vi "Main.vi"(8 "error in (no error)":errorcluster, 11 "ConfocalStage in":refnum<class "ConfocalStage.lvclass">) -> (0 "error out":errorcluster, 3 "component":refnum<class "ConfocalStage.lvclass">)   [LabVIEW 2012, in "ConfocalStage.lvclass"]
doc: "Main VI of the component. This should contain the GUI of your component and be called when creating an executable."
uses:
  ConfocalStage.lvclass
  <vilib>/Distrio/Murmex/Murmex/command_enum.ctl
  <vilib>/Distrio/Murmex/InitialiseMessage/InitialiseMessage.lvclass
  <vilib>/Distrio/Murmex/ConfigureMessage/ConfigureMessage.lvclass
  <vilib>/Distrio/Murmex/TerminateMessage/TerminateMessage.lvclass
  <vilib>/Distrio/Murmex/GenericMessage/GenericMessage.lvclass
  ConfocalStage.lvclass/ConfocalStage.ctl
  <vilib>/Distrio/Murmex/Murmex/Murmex.lvclass
  <vilib>/Distrio/Murmex/Murmex/Set configure at initialise.vi
  <vilib>/Distrio/Murmex/Murmex/Set log reference.vi
  <vilib>/Distrio/Murmex/Murmex/Set VI reference.vi
  <vilib>/Distrio/Murmex/Murmex/Get ID.vi
  <vilib>/Distrio/Murmex/Murmex/Set write log to disk.vi
  <vilib>/Distrio/Murmex/Message/Message.lvclass
panel:
  in  "button:quit":bool
  in  "button:configure":bool
  in  "terminate?":bool
  in  "Tab Control":enum32{"User", "Debug"}(tab)
  in  "focus step":dbl
  in  "Y step":dbl
  in  "X step":dbl
  in  "button:focus_forward":bool
  in  "button:focus_backward":bool
  in  "button:Y_forward":bool
  in  "button:Y_backward":bool
  in  "button:X_forward":bool
  in  "button:X_backward":bool
  in  "button:set as focus max":bool
  in  "button:set as Y max":bool
  in  "button:set as X max":bool
  in  "button:set as focus min":bool
  in  "button:set as Y min":bool
  in  "button:set as X min":bool
  in  "button:set as origin":bool
  in  "X position":dbl
  in  "Y position":dbl
  in  "focus position":dbl
  out "out of limits?":bool
  in  "Component id":string="ConfStage"
  in  "button:send command":bool
  in  "command":T1
  in  "generic command":string
  out "log":string
  # "Position"
  # "Step size"
  # "X"
  # "Y"
  # "Focus"
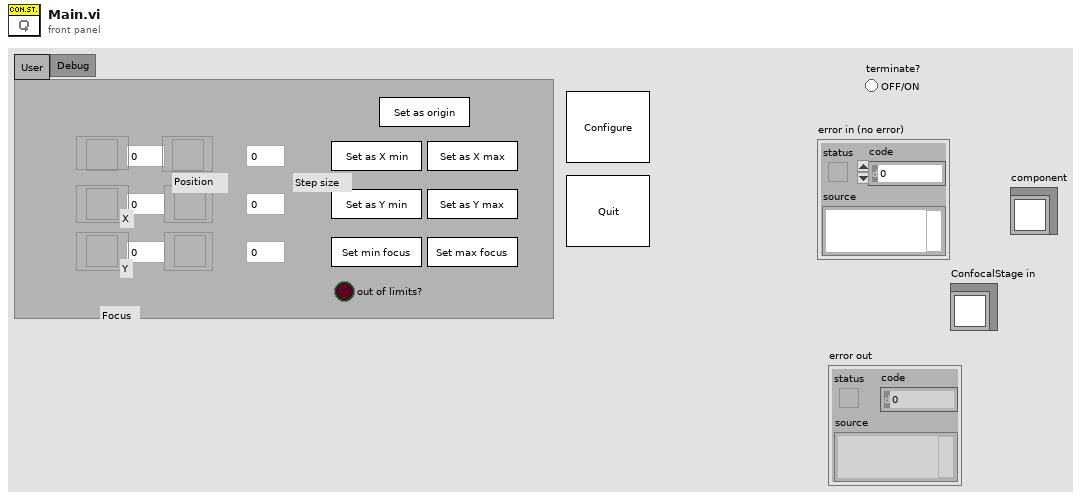
[diagram p1: front panel]
types:
  T1 = typedef "Murmex.lvlib/Murmex.lvclass/command_enum.ctl" = enum16{"null", "initialise", "reset", "terminate", "acknowledge", "update", "inspect", "inform", "proceed", "start", "stop", "fetch", "configure", "generic"}
  T2 = enum8{"Enabled", "Disabled", "Disabled and Grayed Out"}
  T3 = typedef "Murmex.lvclass/command_enum.ctl" = enum16{"null", "initialise", "reset", "terminate", "acknowledge", "update", "inspect", "inform", "proceed", "start", "stop", "fetch", "configure", "generic"}
  T4 = typedef "Murmex.lvclass/Event type enumerations.ctl" = enum16{"before", "after"}
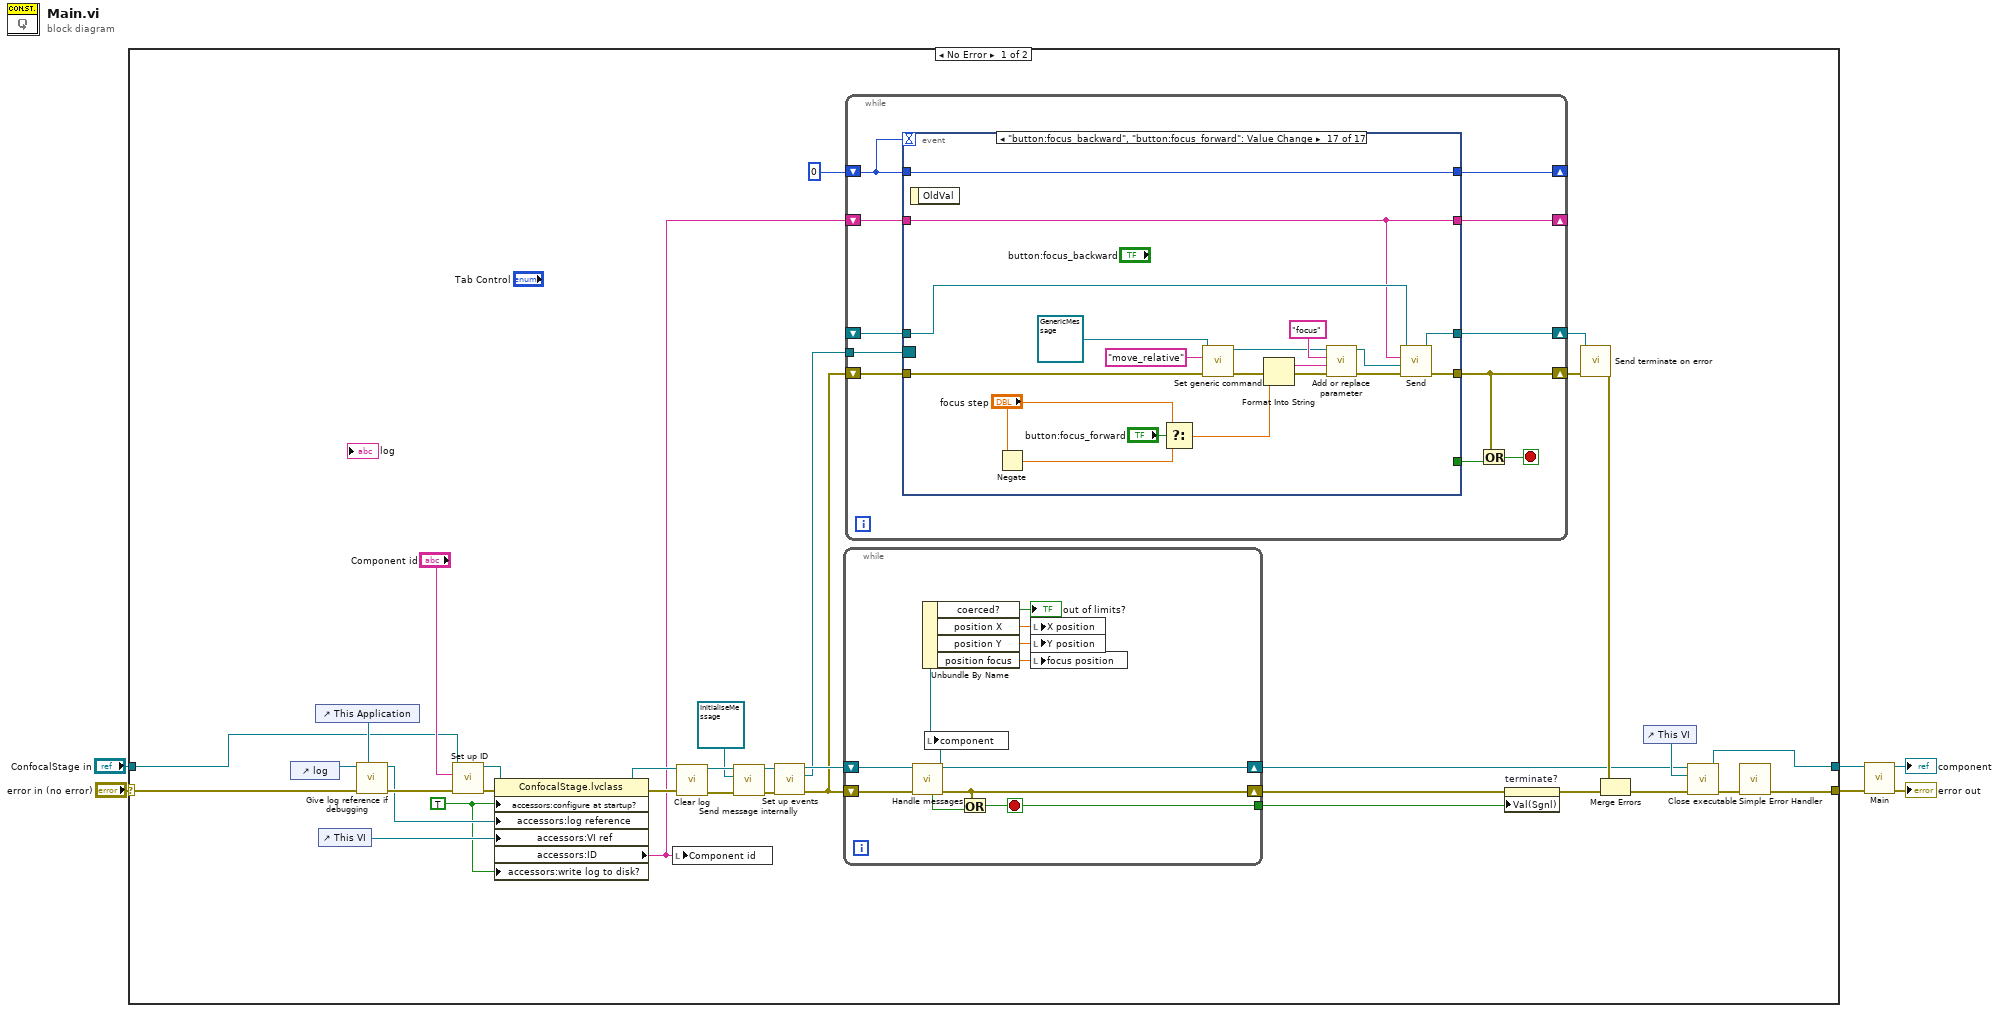
[diagram p0: block diagram]
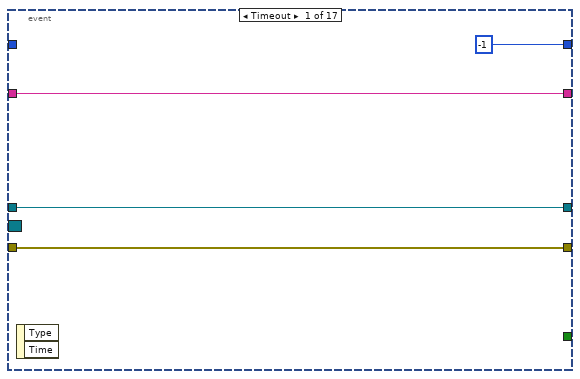
[diagram p2: hidden frame]
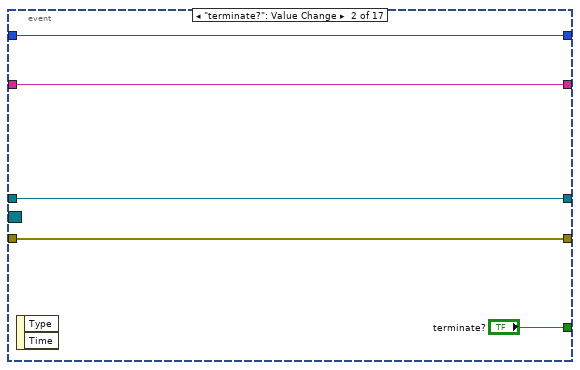
[diagram p3: hidden frame]
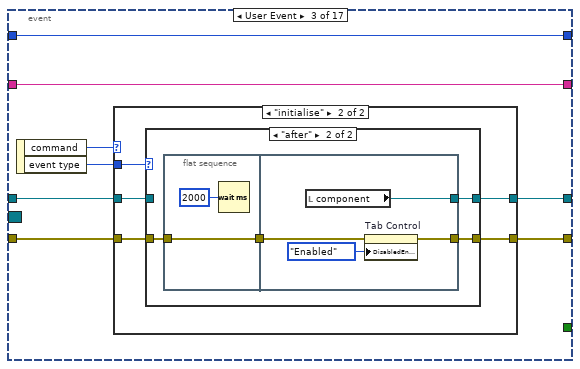
[diagram p4: hidden frame]
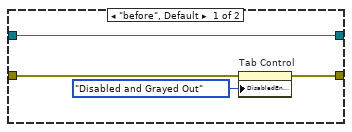
[diagram p6: hidden frame]
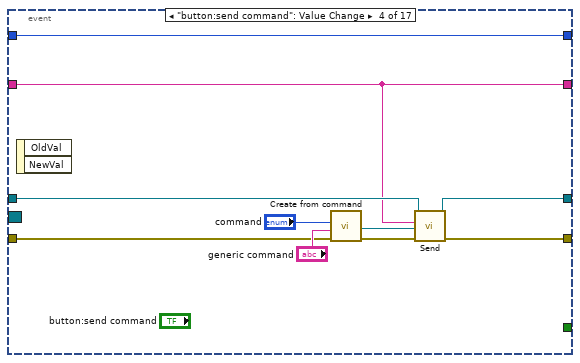
[diagram p7: hidden frame]
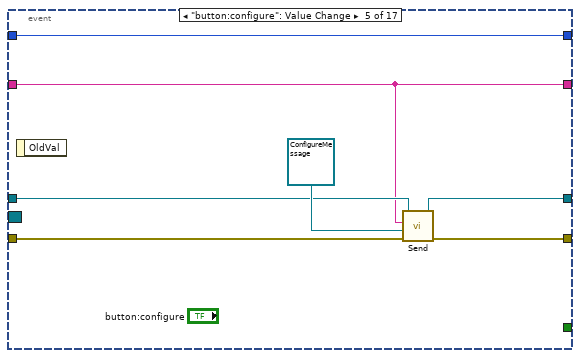
[diagram p8: hidden frame]
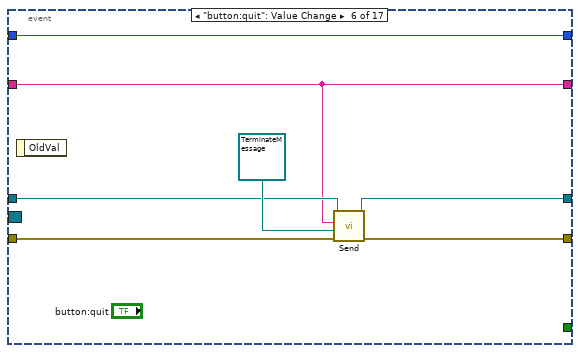
[diagram p9: hidden frame]
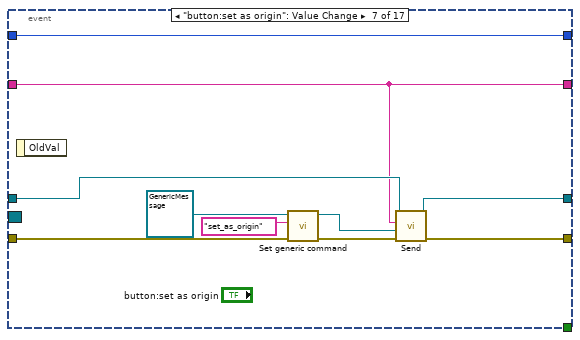
[diagram p10: hidden frame]
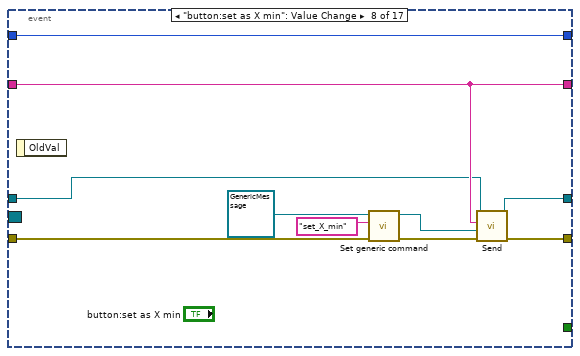
[diagram p11: hidden frame]
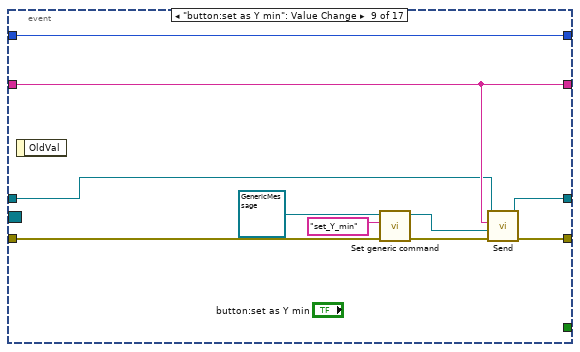
[diagram p12: hidden frame]
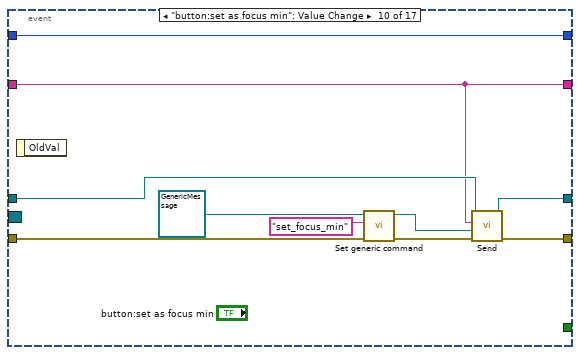
[diagram p13: hidden frame]
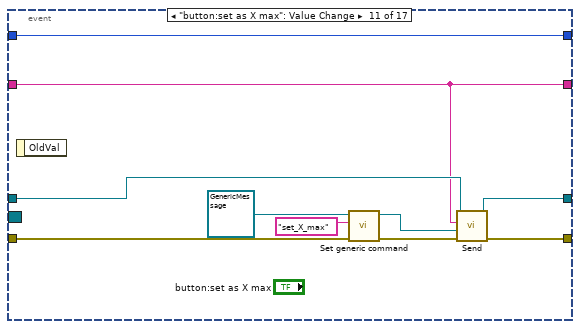
[diagram p14: hidden frame]
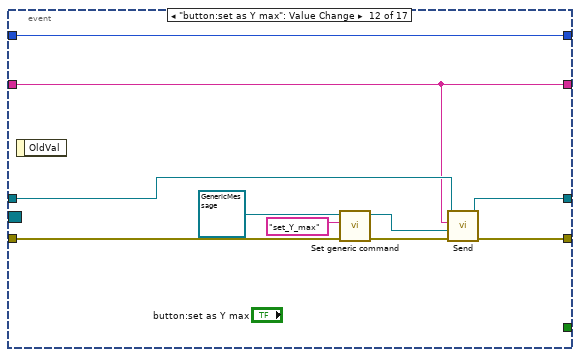
[diagram p15: hidden frame]
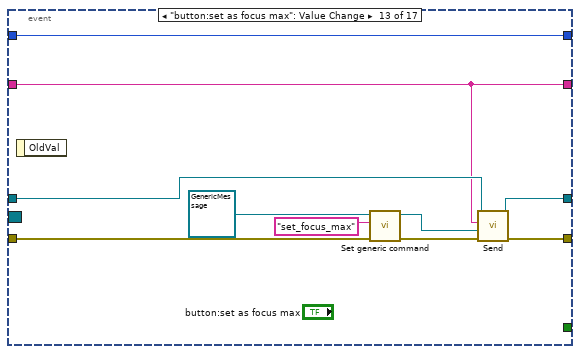
[diagram p16: hidden frame]
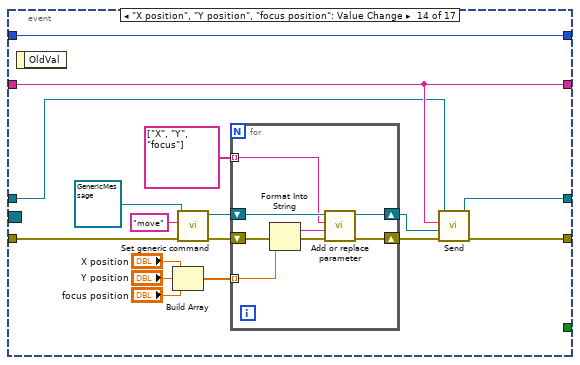
[diagram p17: hidden frame]
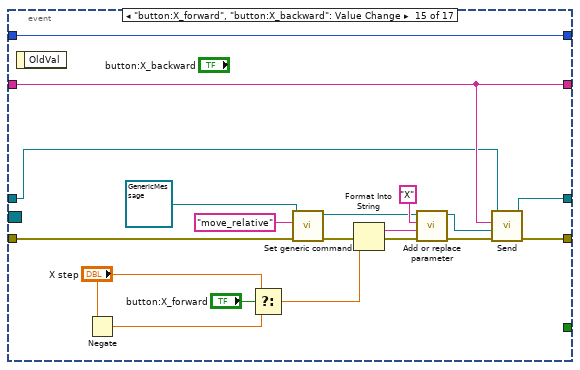
[diagram p18: hidden frame]
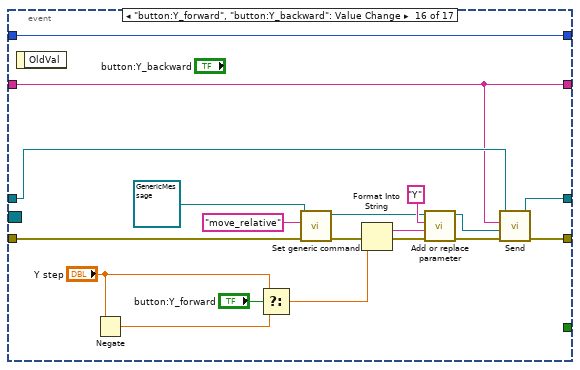
[diagram p19: hidden frame]
diagram:
  n1 = case shown="No Error" "error in (no error)" {
    selector: "error in (no error)" -> [w26 w278]
    tunnel: [w14 w278] -> w3
    tunnel: [w13 w277] -> w2
    tunnel: "ConfocalStage in" -> [w25 w277]
    frame No Error {
      w7 = TRUE ("configure at startup?")
      n2 = control-ref of="log"() -> (w35:refnum<vi>)
      n3 = control-ref of="This Application"() -> (w41:refnum<vi>)
      n4 = control-ref of="This VI"() -> (w34:refnum<vi>)
      n5 = call "Give log reference if debugging.vi"("application ref"=w41, "error in (no error)"=w26, "log reference in"=w35) -> ("error out"=w40:errorcluster, "log reference out"=w36:refnum<vi>)  [unwired: 6 in, 1 out]
      n6 = call <vilib>:"Set up ID.vi"("error in (no error)"=w40, "component ID"="Component id", "MurmexBase in"=w25) -> ("error out"=w38:errorcluster, "MurmexBase out"=w37:refnum<class "ConfocalStage.lvclass">)  [unwired: 6 in, 1 out]
      n7 = property class="ConfocalStage.lvclass"(reference=w37, error in=w38, "accessors:configure at startup?"=w7, "accessors:log reference"=w36, "accessors:VI ref"=w34, "accessors:write log to disk?"=w7) -> (reference out=w27:refnum<class "ConfocalStage.lvclass">, error out=w29:errorcluster, "accessors:ID"=w22:string)
      n8 = local write "Component id"(w22) -> ()
      n9 = call <vilib>:"Clear log.vi"("error in (no error)"=w29, "MurmexBase in"=w27) -> ("error out"=w32:errorcluster, "MurmexBase out"=w33:refnum<class "ConfocalStage.lvclass">)  [unwired: 8 in]
      n10 = call <vilib>:"Send message internally.vi"("error in (no error)"=w32, "Message"=refnum<class "InitialiseMessage.lvclass"> refnum ("InitialiseMessage"), "Murmex in"=w33) -> ("error out"=w31:errorcluster, "Murmex out"=w30:refnum<class "ConfocalStage.lvclass">)  [unwired: 7 in]
      n11 = call <vilib>:"Set up events.vi"("error in (no error)"=w31, "MurmexBase in"=w30) -> ("error out"=w23:errorcluster, "Event Registration Refnum"=w21:refnum<event-registration>, "MurmexBase out"=w24:refnum<class "ConfocalStage.lvclass">)  [unwired: 7 in]
      n12 = while {
        shift-right: [w271] -> w15
        shift-left: w24 -> [w274]
        shift-right: [w273] -> w12
        shift-left: w23 -> [w275]
        tunnel: [w272] -> w10
        stop <- w272 stop-if-true
        n13 = call <vilib>:"Handle messages.vi"("error in (no error)"=w275, "Murmex in"=w274) -> ("error out"=w273:errorcluster, "Murmex out"=w271:refnum<class "ConfocalStage.lvclass">, "terminated?"=w276:bool)  [unwired: 7 in]
        n14 = Unbundle By Name(w271) -> ("coerced?"=→"out of limits?":bool, "position X"=w270:dbl, "position Y"=w269:dbl, "position focus"=w268:dbl)
        n15 = local write "component"(w271) -> ()
        n16 = Or(x=w273, y=w276) -> (x .or. y?=w272:bool)
        n17 = local write "X position"(w270) -> ()
        n18 = local write "Y position"(w269) -> ()
        n19 = local write "focus position"(w268) -> ()
      }
      n20 = while {
        shift-right: [w45] -> w9
        shift-left: w23 -> [w49]
        shift-right: [w48] -> _
        shift-left: w22 -> [w47]
        tunnel: w21 -> [w52]
        shift-right: [w50] -> _
        shift-left: 0 -> [w51]
        shift-right: [w43] -> w8
        shift-left: _ -> [w42]
        stop <- w44 stop-if-true
        n21 = event shown="[16] \"button:focus_backward\", \"button:focus_forward\": Value Change" {
          selector: w52 -> [_ _ _ _ _ _ _ _ _ _ _ _ _ _ _ _ _]
          dyn-events: _ -> [_ _ _ _ _ _ _ _ _ _ _ _ _ _ _ _ _]
          timeout: w51 -> [_ _ _ _ _ _ _ _ _ _ _ _ _ _ _ _ _]
          tunnel: w51 -> [_ w61 w69 w91 w101 w109 w115 w127 w137 w146 w155 w165 w175 w187 w213 w232 w250]
          tunnel: [-1 w61 w69 w91 w101 w109 w115 w127 w137 w146 w155 w165 w175 w187 w213 w232 w250] -> w50
          tunnel: [w55 w59 w65 w95 w105 w112 w120 w129 w139 w149 w159 w169 w180 w190 w215 w236 w254] -> w45
          tunnel: w49 -> [w55 w59 w66 w96 w106 w113 w122 w130 w140 w150 w160 w170 w179 w195 w219 w235 w255]
          tunnel: [w54 w60 w62 w93 w103 w108 w116 w128 w138 w147 w156 w166 w176 w188 w214 w233 w251] -> w48
          tunnel: w47 -> [w54 w60 w62 w93 w103 w108 w116 w128 w138 w147 w156 w166 w176 w188 w214 w233 w251]
          tunnel: [_ "terminate?" _ _ _ _ _ _ _ _ _ _ _ _ _ _ _] -> w46
          tunnel: [w53 w57 w64 w92 w102 w110 w117 w125 w135 w145 w157 w167 w177 w185 w211 w231 w252] -> w43
          tunnel: w42 -> [w53 w57 w63 w94 w104 w111 w118 w126 w136 w148 w158 w168 w178 w186 w212 w234 w253]
          event Timeout {
            n22 = event-data() -> ()  [unwired: 1 in, 2 out]
          }
          event "terminate?": Value Change {
            n23 = event-data() -> ()  [unwired: 1 in, 2 out]
          }
          event User Event {
            n24 = event-data() -> ("command"=w68:T3, "event type"=w67:T4)  [unwired: 1 in]
            n25 = case shown="\"initialise\"" w68 {
              tunnel: w67 -> [_ w76]
              tunnel: w66 -> [w70 w75]
              tunnel: [w70 w74] -> w65
              tunnel: [w71 w73] -> w64
              tunnel: w63 -> [w71 w72]
              frame "null", Default {
              }
              frame "initialise" {
                n26 = case shown="\"after\"" w76 {
                  tunnel: w75 -> [w80 w83]
                  tunnel: [w79 w82] -> w74
                  tunnel: [w77 w81] -> w73
                  tunnel: w72 -> [w77 _]
                  frame "before", Default {
                    n27 = property on="Tab Control" class="TabCtl (strict)"(error in=w80, "DisabledEnum"=T2."Disabled and Grayed Out" ("Disabled")) -> (error out=w79:errorcluster)  [unwired: 1 in, 1 out]
                  }
                  frame "after" {
                    n28 = flat-sequence {
                      tunnel: [w85] -> w84
                      tunnel: w83 -> [w85]
                      tunnel: w84 -> [w89]
                      tunnel: [w88] -> w82
                      tunnel: [w87] -> w81
                      frame #0 {
                        n29 = Wait (ms)(milliseconds to wait=u32 2000) -> ()  [unwired: 1 out]
                      }
                      frame #1 {
                        n30 = local read "component"() -> (w87:refnum<class "ConfocalStage.lvclass">)
                        n31 = property on="Tab Control" class="TabCtl (strict)"(error in=w89, "DisabledEnum"=T2."Enabled" ("Disabled")) -> (error out=w88:errorcluster)  [unwired: 1 in, 1 out]
                      }
                    }
                  }
                }
              }
            }
          }
          event "button:send command": Value Change {
            n32 = event-data() -> ()  [unwired: 1 in, 2 out]
            n33 = call <vilib>:"Create from command.vi"("error in (no error)"=w96, "generic command"="generic command", "command"="command") -> ("error out"=w97:errorcluster, "Message out"=w100:refnum<class "Message.lvclass">)  [unwired: 7 in]
            n34 = call <vilib>:"Send.vi"("error in (no error)"=w97, "Message"=w100, "recipient"=w93, "Murmex in"=w94) -> ("error out"=w95:errorcluster, "Murmex out"=w92:refnum<class "ConfocalStage.lvclass">)  [unwired: 6 in]
          }
          event "button:configure": Value Change {
            n35 = event-data() -> ()  [unwired: 1 in, 1 out]
            n36 = call <vilib>:"Send.vi"("error in (no error)"=w106, "Message"=refnum<class "ConfigureMessage.lvclass"> refnum ("ConfigureMessage"), "recipient"=w103, "Murmex in"=w104) -> ("error out"=w105:errorcluster, "Murmex out"=w102:refnum<class "ConfocalStage.lvclass">)  [unwired: 6 in]
          }
          event "button:quit": Value Change {
            n37 = event-data() -> ()  [unwired: 1 in, 1 out]
            n38 = call <vilib>:"Send.vi"("error in (no error)"=w113, "Message"=refnum<class "TerminateMessage.lvclass"> refnum ("TerminateMessage"), "recipient"=w108, "Murmex in"=w111) -> ("error out"=w112:errorcluster, "Murmex out"=w110:refnum<class "ConfocalStage.lvclass">)  [unwired: 6 in]
          }
          event "button:set as origin": Value Change {
            n39 = event-data() -> ()  [unwired: 1 in, 1 out]
            n40 = call <vilib>:"Set generic command.vi"("error in (no error)"=w122, "generic command"="set_as_origin", "GenericMessage in"=refnum<class "GenericMessage.lvclass"> refnum ("Message in")) -> ("error out"=w121:errorcluster, "GenericMessage out"=w119:refnum<class "GenericMessage.lvclass">)  [unwired: 7 in]
            n41 = call <vilib>:"Send.vi"("error in (no error)"=w121, "Message"=w119, "recipient"=w116, "Murmex in"=w118) -> ("error out"=w120:errorcluster, "Murmex out"=w117:refnum<class "ConfocalStage.lvclass">)  [unwired: 6 in]
          }
          event "button:set as X min": Value Change {
            n42 = event-data() -> ()  [unwired: 1 in, 1 out]
            n43 = call <vilib>:"Set generic command.vi"("error in (no error)"=w130, "generic command"="set_X_min", "GenericMessage in"=refnum<class "GenericMessage.lvclass"> refnum ("Message in")) -> ("error out"=w133:errorcluster, "GenericMessage out"=w134:refnum<class "GenericMessage.lvclass">)  [unwired: 7 in]
            n44 = call <vilib>:"Send.vi"("error in (no error)"=w133, "Message"=w134, "recipient"=w128, "Murmex in"=w126) -> ("error out"=w129:errorcluster, "Murmex out"=w125:refnum<class "ConfocalStage.lvclass">)  [unwired: 6 in]
          }
          event "button:set as Y min": Value Change {
            n45 = event-data() -> ()  [unwired: 1 in, 1 out]
            n46 = call <vilib>:"Set generic command.vi"("error in (no error)"=w140, "generic command"="set_Y_min", "GenericMessage in"=refnum<class "GenericMessage.lvclass"> refnum ("Message in")) -> ("error out"=w142:errorcluster, "GenericMessage out"=w141:refnum<class "GenericMessage.lvclass">)  [unwired: 7 in]
            n47 = call <vilib>:"Send.vi"("error in (no error)"=w142, "Message"=w141, "recipient"=w138, "Murmex in"=w136) -> ("error out"=w139:errorcluster, "Murmex out"=w135:refnum<class "ConfocalStage.lvclass">)  [unwired: 6 in]
          }
          event "button:set as focus min": Value Change {
            n48 = event-data() -> ()  [unwired: 1 in, 1 out]
            n49 = call <vilib>:"Set generic command.vi"("error in (no error)"=w150, "generic command"="set_focus_min", "GenericMessage in"=refnum<class "GenericMessage.lvclass"> refnum ("Message in")) -> ("error out"=w152:errorcluster, "GenericMessage out"=w151:refnum<class "GenericMessage.lvclass">)  [unwired: 7 in]
            n50 = call <vilib>:"Send.vi"("error in (no error)"=w152, "Message"=w151, "recipient"=w147, "Murmex in"=w148) -> ("error out"=w149:errorcluster, "Murmex out"=w145:refnum<class "ConfocalStage.lvclass">)  [unwired: 6 in]
          }
          event "button:set as X max": Value Change {
            n51 = event-data() -> ()  [unwired: 1 in, 1 out]
            n52 = call <vilib>:"Set generic command.vi"("error in (no error)"=w160, "generic command"="set_X_max", "GenericMessage in"=refnum<class "GenericMessage.lvclass"> refnum ("Message in")) -> ("error out"=w162:errorcluster, "GenericMessage out"=w161:refnum<class "GenericMessage.lvclass">)  [unwired: 7 in]
            n53 = call <vilib>:"Send.vi"("error in (no error)"=w162, "Message"=w161, "recipient"=w156, "Murmex in"=w158) -> ("error out"=w159:errorcluster, "Murmex out"=w157:refnum<class "ConfocalStage.lvclass">)  [unwired: 6 in]
          }
          event "button:set as Y max": Value Change {
            n54 = event-data() -> ()  [unwired: 1 in, 1 out]
            n55 = call <vilib>:"Set generic command.vi"("error in (no error)"=w170, "generic command"="set_Y_max", "GenericMessage in"=refnum<class "GenericMessage.lvclass"> refnum ("Message in")) -> ("error out"=w172:errorcluster, "GenericMessage out"=w171:refnum<class "GenericMessage.lvclass">)  [unwired: 7 in]
            n56 = call <vilib>:"Send.vi"("error in (no error)"=w172, "Message"=w171, "recipient"=w166, "Murmex in"=w168) -> ("error out"=w169:errorcluster, "Murmex out"=w167:refnum<class "ConfocalStage.lvclass">)  [unwired: 6 in]
          }
          event "button:set as focus max": Value Change {
            n57 = event-data() -> ()  [unwired: 1 in, 1 out]
            n58 = call <vilib>:"Set generic command.vi"("error in (no error)"=w179, "generic command"="set_focus_max", "GenericMessage in"=refnum<class "GenericMessage.lvclass"> refnum ("Message in")) -> ("error out"=w182:errorcluster, "GenericMessage out"=w181:refnum<class "GenericMessage.lvclass">)  [unwired: 7 in]
            n59 = call <vilib>:"Send.vi"("error in (no error)"=w182, "Message"=w181, "recipient"=w176, "Murmex in"=w178) -> ("error out"=w180:errorcluster, "Murmex out"=w177:refnum<class "ConfocalStage.lvclass">)  [unwired: 6 in]
          }
          event "X position", "Y position", "focus position": Value Change {
            n60 = event-data() -> ()  [unwired: 1 in, 1 out]
            n61 = Build Array("X position", "Y position", "focus position") -> (w198:dbl[])
            n62 = call <vilib>:"Set generic command.vi"("error in (no error)"=w195, "generic command"="move", "GenericMessage in"=refnum<class "GenericMessage.lvclass"> refnum ("Message in")) -> ("error out"=w194:errorcluster, "GenericMessage out"=w193:refnum<class "GenericMessage.lvclass">)  [unwired: 7 in]
            n63 = for {
              tunnel: w198 -> [w203] mode=indexing
              shift-right: [w204] -> w191
              shift-left: w194 -> [w208]
              shift-right: [w205] -> w189
              shift-left: w193 -> [w206]
              tunnel: string[] ["X", "Y", "focus"] -> [w202] mode=indexing
              n64 = Format Into String(error in=w208, w203) -> (resulting string=w209:string, error out=w207:errorcluster)  [unwired: 2 in]
              n65 = call <vilib>:"Add or replace parameter.vi"("error in (no error)"=w207, "value"=w209, "name"=w202, "Message in"=w206) -> ("error out"=w204:errorcluster, "Message out"=w205:refnum<class "GenericMessage.lvclass">)  [unwired: 6 in]
            }
            n66 = call <vilib>:"Send.vi"("error in (no error)"=w191, "Message"=w189, "recipient"=w188, "Murmex in"=w186) -> ("error out"=w190:errorcluster, "Murmex out"=w185:refnum<class "ConfocalStage.lvclass">)  [unwired: 6 in]
          }
          event "button:X_forward", "button:X_backward": Value Change {
            n67 = event-data() -> ()  [unwired: 1 in, 1 out]
            n68 = Negate(x="X step") -> (-x=w226:dbl)
            n69 = Select(t="X step", s="button:X_forward", f=w226) -> (s? t:f=w210:dbl)
            n70 = call <vilib>:"Set generic command.vi"("error in (no error)"=w219, "generic command"="move_relative", "GenericMessage in"=refnum<class "GenericMessage.lvclass"> refnum ("Message in")) -> ("error out"=w218:errorcluster, "GenericMessage out"=w221:refnum<class "GenericMessage.lvclass">)  [unwired: 7 in]
            n71 = Format Into String(error in=w218, w210) -> (resulting string=w222:string, error out=w217:errorcluster)  [unwired: 2 in]
            n72 = call <vilib>:"Add or replace parameter.vi"("error in (no error)"=w217, "value"=w222, "name"="X", "Message in"=w221) -> ("error out"=w216:errorcluster, "Message out"=w220:refnum<class "GenericMessage.lvclass">)  [unwired: 6 in]
            n73 = call <vilib>:"Send.vi"("error in (no error)"=w216, "Message"=w220, "recipient"=w214, "Murmex in"=w212) -> ("error out"=w215:errorcluster, "Murmex out"=w211:refnum<class "ConfocalStage.lvclass">)  [unwired: 6 in]
          }
          event "button:Y_forward", "button:Y_backward": Value Change {
            n74 = event-data() -> ()  [unwired: 1 in, 1 out]
            n75 = Negate(x="Y step") -> (-x=w247:dbl)
            n76 = Select(t="Y step", s="button:Y_forward", f=w247) -> (s? t:f=w237:dbl)
            n77 = call <vilib>:"Set generic command.vi"("error in (no error)"=w235, "generic command"="move_relative", "GenericMessage in"=refnum<class "GenericMessage.lvclass"> refnum ("Message in")) -> ("error out"=w240:errorcluster, "GenericMessage out"=w242:refnum<class "GenericMessage.lvclass">)  [unwired: 7 in]
            n78 = Format Into String(error in=w240, w237) -> (resulting string=w243:string, error out=w239:errorcluster)  [unwired: 2 in]
            n79 = call <vilib>:"Add or replace parameter.vi"("error in (no error)"=w239, "value"=w243, "name"="Y", "Message in"=w242) -> ("error out"=w238:errorcluster, "Message out"=w241:refnum<class "GenericMessage.lvclass">)  [unwired: 6 in]
            n80 = call <vilib>:"Send.vi"("error in (no error)"=w238, "Message"=w241, "recipient"=w233, "Murmex in"=w234) -> ("error out"=w236:errorcluster, "Murmex out"=w231:refnum<class "ConfocalStage.lvclass">)  [unwired: 6 in]
          }
          event "button:focus_backward", "button:focus_forward": Value Change {
            n81 = event-data() -> ()  [unwired: 1 in, 1 out]
            n82 = Negate(x="focus step") -> (-x=w266:dbl)
            n83 = Select(t="focus step", s="button:focus_forward", f=w266) -> (s? t:f=w256:dbl)
            n84 = call <vilib>:"Set generic command.vi"("error in (no error)"=w255, "generic command"="move_relative", "GenericMessage in"=refnum<class "GenericMessage.lvclass"> refnum ("Message in")) -> ("error out"=w259:errorcluster, "GenericMessage out"=w261:refnum<class "GenericMessage.lvclass">)  [unwired: 7 in]
            n85 = Format Into String(error in=w259, w256) -> (resulting string=w262:string, error out=w258:errorcluster)  [unwired: 2 in]
            n86 = call <vilib>:"Add or replace parameter.vi"("error in (no error)"=w258, "value"=w262, "name"="focus", "Message in"=w261) -> ("error out"=w257:errorcluster, "Message out"=w260:refnum<class "GenericMessage.lvclass">)  [unwired: 6 in]
            n87 = call <vilib>:"Send.vi"("error in (no error)"=w257, "Message"=w260, "recipient"=w251, "Murmex in"=w253) -> ("error out"=w254:errorcluster, "Murmex out"=w252:refnum<class "ConfocalStage.lvclass">)  [unwired: 6 in]
          }
        }
        n88 = Or(x=w45, y=w46) -> (x .or. y?=w44:bool)
      }
      n89 = property on="terminate?" class="Bool (strict)"(error in=w12, "Val(Sgnl)"=w10) -> (error out=w11:errorcluster)  [unwired: 1 in, 1 out]
      n90 = call <vilib>:"Send terminate on error.vi"("error in (no error)"=w9, "Murmex in"=w8) -> ("error out"=w19:errorcluster)  [unwired: 8 in, 1 out]
      n91 = Merge Errors(w19, w11) -> (w17:errorcluster)
      n92 = control-ref of="This VI"() -> (w18:refnum<vi>)
      n93 = call <vilib>:"Close executable.vi"("error in (no error)"=w17, "main VI ref (optional)"=w18, "MurmexBase in"=w15) -> ("error out"=w16:errorcluster, "MurmexBase out"=w13:refnum<class "ConfocalStage.lvclass">)  [unwired: 7 in]
      n94 = call <vilib>:"Simple Error Handler.vi"("error in (no error)"=w16) -> ("error out"=w14:errorcluster)  [unwired: 4 in, 4 out]
    }
    frame Error {
    }
  }
  n95 = call-parent "Main.vi"("error in (no error)"=w3, "Murmex in"=w2) -> ("error out"=→"error out":errorcluster, "Murmex out"=→"component":refnum<class "ConfocalStage.lvclass">)  [unwired: 8 in]
